vi "write_ini.vi"(8 "error in (no error)":errorcluster caption="错误输入（无错误）", 9 "section name":string, 10 "file ref in":T1, 11 "OneMotion 输入":refnum<class "OneMotion.lvclass">) -> (0 "error out":errorcluster caption="错误输出", 2 "file ref out":T1, 3 "OneMotion 输出":refnum<class "OneMotion.lvclass">)   [LabVIEW 2016, in "MotionControl.lvlib" / "OneMotion.lvclass"]
uses:
  <userlib>/MotionControl/OneMotion/OneMotion.lvclass
  <vilib>/Utility/config.llb/Config Data RefNum.ctl
  <userlib>/MotionControl/OneMotion/OneMotion.lvclass/OneMotion.ctl
  <vilib>/Utility/config.llb/Write Key (String).vi
  <vilib>/Utility/config.llb/Write Key (I32).vi
  <vilib>/Utility/config.llb/Write Key (Double).vi
  <vilib>/Utility/config.llb/Write Key (U32).vi
  <vilib>/Utility/error.llb/Error Cluster From Error Code.vi
  <vilib>/ErrorRing/Error Ring.xnode
  <userlib>/MotionControl/StepMotor/StepMotor.lvclass
  <userlib>/MotionControl/LimitSwitch/LimitSwitch.lvclass
  <vilib>/Utility/config.llb/NI_LVConfig.lvlib
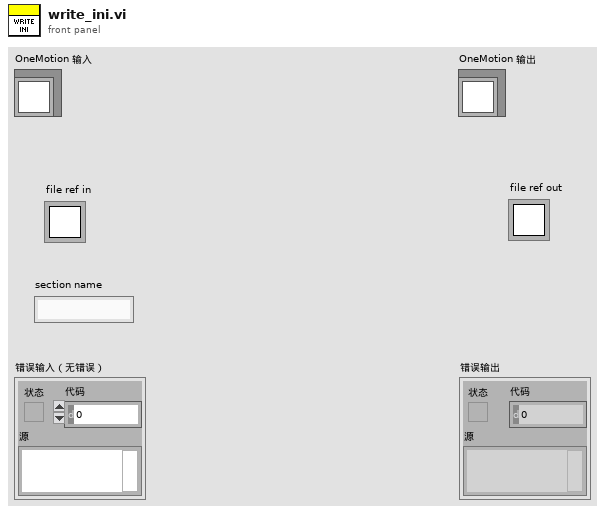
[diagram p1: front panel]
types:
  T1 = typedef "NI_LVConfig.lvlib/Config Data RefNum.ctl" = refnum<k1>
  T2 = typedef "MotionControl.lvlib/OneMotion.lvclass/hard limit option.ctl" = enum16{"STOP, and a 0.5s timeout constraint in move", "STOP, and move disabled"}
  T3 = typedef "MotionControl.lvlib/OneMotion.lvclass/unit mode.ctl" = enum16{"motor (pulse)", "linear (mm) or radial (degree)"}
  T4 = typedef "MotionControl.lvlib/OneMotion.lvclass/backlash option.ctl" = enum16{"no backlash compensation", "compensation: from - to +", "compensation: from + to -"}
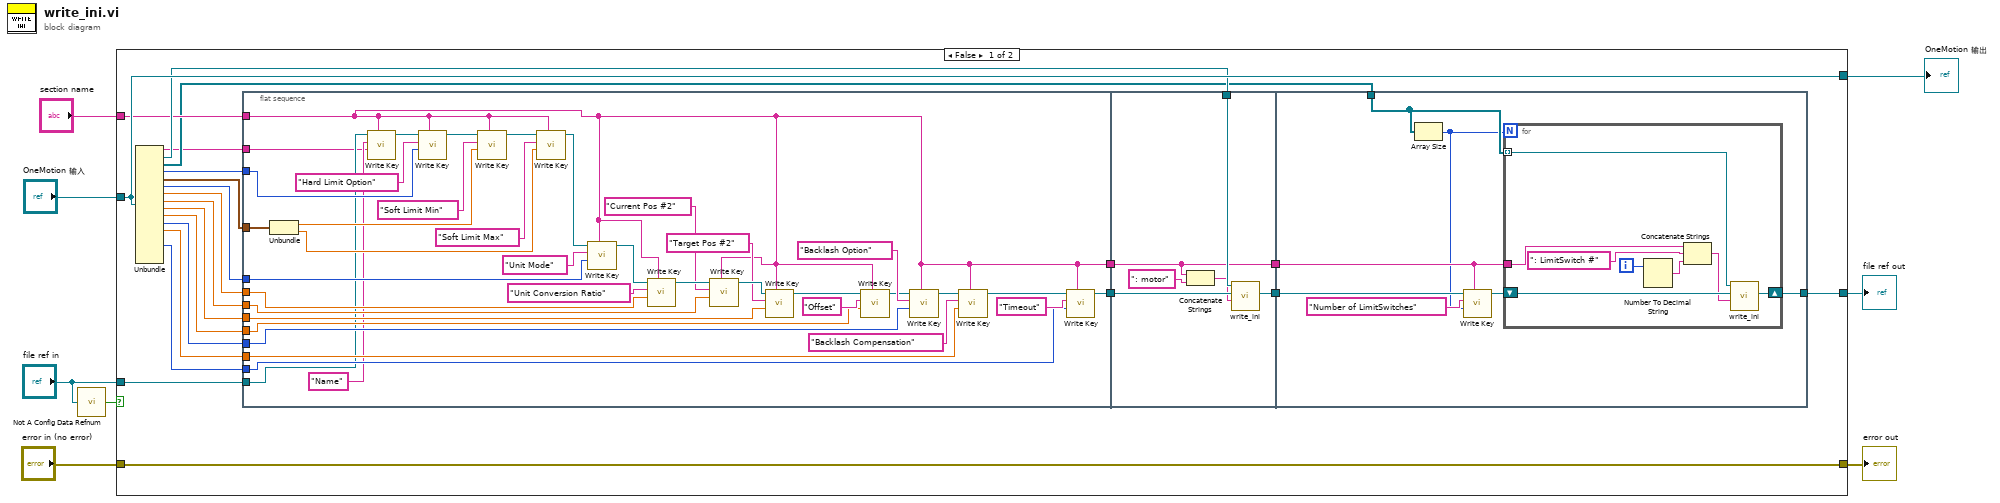
[diagram p0: block diagram]
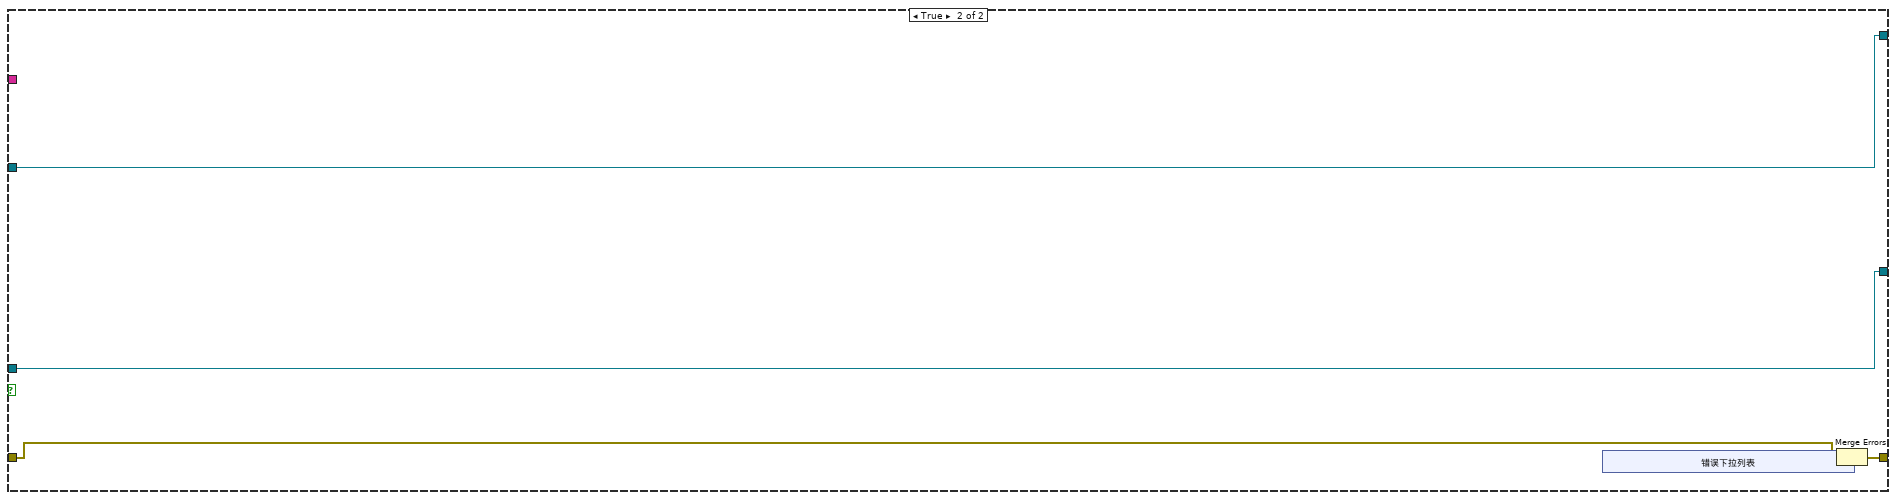
[diagram p2: hidden frame]
diagram:
  n1 = call <vilib>:"Not A Config Data Refnum.vi"("refnum"="file ref in") -> ("not a config data refnum"=w2:bool)
  n2 = case shown="False" w2 {
    tunnel: [w30 w91] -> w8
    tunnel: [w27 w95] -> w6
    tunnel: "OneMotion 输入" -> [w27 w95]
    tunnel: "error in (no error)" -> [w30 w92]
    tunnel: "file ref in" -> [w29 w94]
    tunnel: [w28 w94] -> w3
    tunnel: "section name" -> [w25 _]
    frame False {
      n3 = Unbundle(w27) -> (w10:string, w26:refnum<class "StepMotor.lvclass">, w15:refnum<class "LimitSwitch.lvclass">[], w23:T2, w22:cluster{"min":dbl, "max":dbl}, w21:T3, w20:dbl, w19:dbl, w18:dbl, w11:dbl, w12:T4, w13:dbl, w9:u32)  [unwired: 3 out]
      n4 = flat-sequence {
        tunnel: w29 -> [w33]
        tunnel: w25 -> [w34]
        tunnel: [w50] -> w24
        tunnel: w23 -> [w68]
        tunnel: w22 -> [w49]
        tunnel: w21 -> [w46]
        tunnel: w20 -> [w45]
        tunnel: w19 -> [w44]
        tunnel: w18 -> [w43]
        tunnel: w12 -> [w42]
        tunnel: w13 -> [w41]
        tunnel: w9 -> [w40]
        tunnel: [w34] -> w17
        tunnel: w11 -> [w36]
        tunnel: w10 -> [w31]
        tunnel: w26 -> [w74]
        tunnel: w24 -> [w73]
        tunnel: w17 -> [w70]
        tunnel: [w75] -> w16
        tunnel: [w70] -> w14
        tunnel: [w82] -> w28
        tunnel: w16 -> [w80]
        tunnel: w15 -> [w77]
        tunnel: w14 -> [w81]
        frame #0 {
          n5 = Unbundle(w49) -> ("min"=w48:dbl, "max"=w47:dbl)
          n6 = call-poly <vilib>:"Write Key.vi"("section"=w34, "value"=w31, "key"="Name", "refnum"=w33) -> ("refnum out"=w32:T1)  [unwired: 5 in, 2 out]
          n7 = call-poly <vilib>:"Write Key.vi"("section"=w34, "value"=w68, "key"="Hard Limit Option", "refnum"=w32) -> ("refnum out"=w67:T1)  [unwired: 5 in, 2 out]
          n8 = call-poly <vilib>:"Write Key.vi"("section"=w34, "value"=w48, "key"="Soft Limit Min", "refnum"=w67) -> ("refnum out"=w66:T1)  [unwired: 5 in, 2 out]
          n9 = call-poly <vilib>:"Write Key.vi"("section"=w34, "value"=w47, "key"="Soft Limit Max", "refnum"=w66) -> ("refnum out"=w63:T1)  [unwired: 5 in, 2 out]
          n10 = call-poly <vilib>:"Write Key.vi"("section"=w34, "value"=w46, "key"="Unit Mode", "refnum"=w63) -> ("refnum out"=w62:T1)  [unwired: 5 in, 2 out]
          n11 = call-poly <vilib>:"Write Key.vi"("section"=w34, "value"=w45, "key"="Unit Conversion Ratio", "refnum"=w62) -> ("refnum out"=w61:T1)  [unwired: 5 in, 2 out]
          n12 = call-poly <vilib>:"Write Key.vi"("section"=w34, "value"=w44, "key"="Current Pos #2", "refnum"=w61) -> ("refnum out"=w57:T1)  [unwired: 5 in, 2 out]
          n13 = call-poly <vilib>:"Write Key.vi"("section"=w34, "value"=w43, "key"="Target Pos #2", "refnum"=w57) -> ("refnum out"=w39:T1)  [unwired: 5 in, 2 out]
          n14 = call-poly <vilib>:"Write Key.vi"("section"=w34, "value"=w36, "key"="Offset", "refnum"=w39) -> ("refnum out"=w38:T1)  [unwired: 5 in, 2 out]
          n15 = call-poly <vilib>:"Write Key.vi"("section"=w34, "value"=w42, "key"="Backlash Option", "refnum"=w38) -> ("refnum out"=w56:T1)  [unwired: 5 in, 2 out]
          n16 = call-poly <vilib>:"Write Key.vi"("section"=w34, "value"=w41, "key"="Backlash Compensation", "refnum"=w56) -> ("refnum out"=w52:T1)  [unwired: 5 in, 2 out]
          n17 = call-poly <vilib>:"Write Key.vi"("section"=w34, "value"=w40, "key"="Timeout", "refnum"=w52) -> ("refnum out"=w50:T1)  [unwired: 5 in, 2 out]
        }
        frame #1 {
          n18 = Concatenate Strings(w70, ": motor") -> (w71:string)
          n19 = call-dynamic "write_ini.vi"("section name"=w71, "file ref in"=w73, "StepMotor 输入"=w74) -> ("file ref out"=w75:T1)  [unwired: 6 in, 2 out]
        }
        frame #2 {
          n20 = Array Size(array=w77) -> (size(s)=w76:i32)
          n21 = call-poly <vilib>:"Write Key.vi"("section"=w81, "value"=w76, "key"="Number of LimitSwitches", "refnum"=w80) -> ("refnum out"=w79:T1)  [unwired: 5 in, 2 out]
          n22 = for {
            N: w76 -> [_]
            tunnel: w77 -> [w90] mode=indexing
            shift-right: [w88] -> w82
            shift-left: w79 -> [w89]
            tunnel: w81 -> [w86]
            i -> [w85]
            n23 = Number To Decimal String(number=w85) -> (decimal integer string=w84:string)  [unwired: 1 in]
            n24 = Concatenate Strings(w86, ": LimitSwitch #", w84) -> (w83:string)
            n25 = call-dynamic "write_ini.vi"("section name"=w83, "file ref in"=w89, "LimitSwitch 输入"=w90) -> ("file ref out"=w88:T1)  [unwired: 6 in, 2 out]
          }
        }
      }
    }
    frame True {
      n26 = xnode "错误下拉列表"() -> ("error out"=w93:errorcluster)
      n27 = Merge Errors(w92, w93) -> (w91:errorcluster)
    }
  }
  "error out" <- w8
  "OneMotion 输出" <- w6
  "file ref out" <- w3
